vi "Pre Launch Init.vi"(11 "WS Server in":refnum<class "WS Server.lvclass">) -> (0 "error out":errorcluster, 3 "WS Server out":refnum<class "WS Server.lvclass">)   [LabVIEW 2016, in "WebSocket Networking.lvlib" / "WS Server.lvclass"]
doc: "--\nCopyright © 2017 Composed SystemsI All rights reserved.\n\nAuthor: Jon McBee <jon.mcbee@composed.io>\n\nThis library is provided \"AS IS\" ,WITHOUT WARRANTIES OR\nCONDITIONS OF ANY KIND, either express or implied.\n\nComposed Systems -- composed.io\n\nStream 0.0.1.1\nJon McBee - Composed Systems\nCopyright (c) 2017, Composed Systems"
uses:
  <userlib>/Common Components/WebSocket Networking/WS Server/WS Server.lvclass
  C:/Program Files (x86)/National Instruments/LabVIEW 2016/user.lib/Composed Systems/Stream/Mediator/Classes/Mediated Asynchronous Actor/Mediated Asynchronous Actor.lvclass
  C:/Program Files (x86)/National Instruments/LabVIEW 2016/user.lib/Composed Systems/Stream/Mediator/Classes/Websocket Server Actor/Websocket Server/Websocket Server.lvclass
  <userlib>/Common Components/WebSocket Networking/WS Client/WS Client.lvclass
  C:/Program Files (x86)/National Instruments/LabVIEW 2016/user.lib/Composed Systems/Stream/Mediator/Classes/Websocket Client Handler Actor/Websocket Client Handler/Websocket Client Handler.lvclass
  <userlib>/Composed Systems/Stream/Mediator/Classes/Websocket Server Actor/Websocket Server/Websocket Server.lvclass/Websocket Server.ctl
  <userlib>/Common Components/WebSocket Networking/WS Client/WS Client.lvclass/WS Client.ctl
  <userlib>/Composed Systems/Stream/Mediator/Classes/Websocket Server Actor/Websocket Server/Websocket Server.lvclass
  <userlib>/Composed Systems/Stream/Mediator/Classes/Mediated Asynchronous Actor/Mediated Asynchronous Actor.lvclass
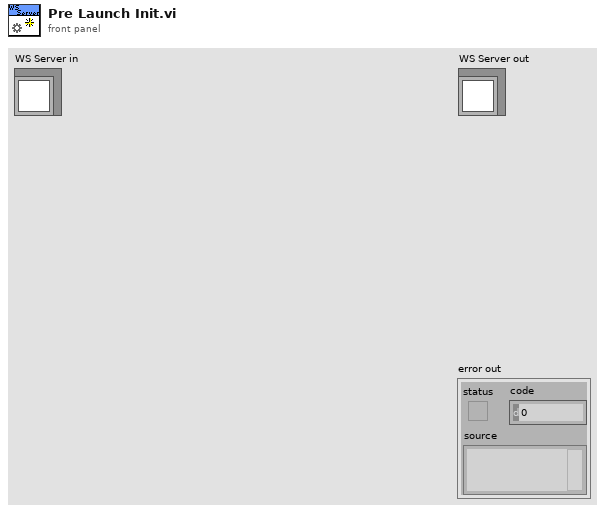
[diagram p1: front panel]
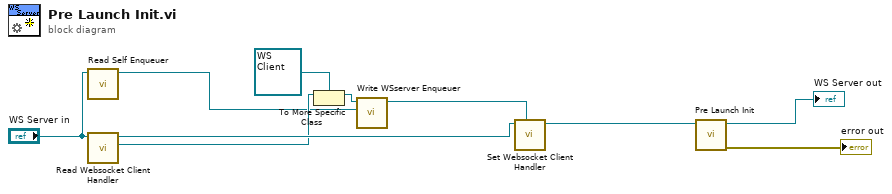
[diagram p0: block diagram]
diagram:
  n1 = call <userlib>:"Read Self Enqueuer.vi"("Mediated Asynchronous Actor in"="WS Server in") -> ("Self Enqueuer"=w3:refnum<class "Message Transport Queue.lvclass">)  [unwired: 10 in]
  n2 = call <userlib>:"Read Websocket Client Handler.vi"("Websocket Server in"="WS Server in") -> ("Stream Mediator.lvlib:Websocket Client Handler.lvclass"=w7:refnum<class "Websocket Client Handler.lvclass">, "Websocket Server out"=w8:refnum<class "WS Server.lvclass">)  [unwired: 9 in]
  n3 = To More Specific Class(target class=refnum<class "WS Client.lvclass"> refnum ("WebSocket Networking.lvlib:WS Client.lvclass"), reference=w7) -> (specific class reference=w6:refnum<class "WS Client.lvclass">)  [unwired: 1 in, 1 out]
  n4 = call <userlib>:"Write WSserver Enqueuer.vi"("Stream Mediator.lvlib:Message Transport Queue.lvclass"=w3, "WS Client in"=w6) -> ("WS Client out"=w1:refnum<class "WS Client.lvclass">)  [unwired: 9 in]
  n5 = call <userlib>:"Set Websocket Client Handler.vi"("Websocket Client Handler"=w1, "Websocket Server in"=w8) -> ("Websocket Server out"=w2:refnum<class "WS Server.lvclass">)  [unwired: 8 in, 1 out]
  n6 = call-parent "Pre Launch Init.vi"("Websocket Server in"=w2) -> ("error out"=→"error out":errorcluster, "Websocket Server out"=→"WS Server out":refnum<class "WS Server.lvclass">)  [unwired: 9 in]
